vi "Setpoint Status.vi"(8 "error in (no error)":errorcluster, 10 "Output (1:1)":u16(ring)=1 items=["1"=1, "2"=2], 11 "VISA resource name":refnum<visa-resource-name>) -> (0 "error out":errorcluster, 2 "Setpoint":dbl format="%.4f", 3 "VISA resource name out":refnum<visa-resource-name>)   [LabVIEW 2014, in "Lake Shore 335.lvlib"]
doc: "Returns the setpoint value for the selected output."
uses:
  Lake Shore 335.lvlib
  Instance           1 23Saved   Setpoint Status .vi
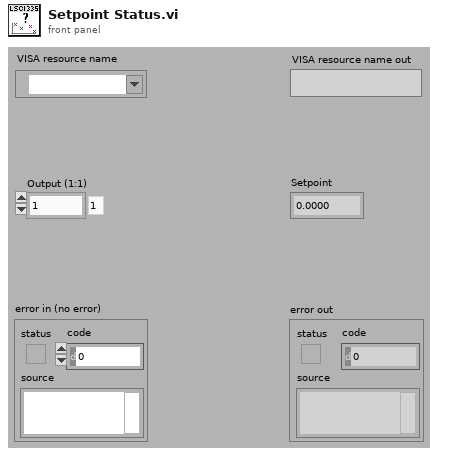
[diagram p1: front panel]
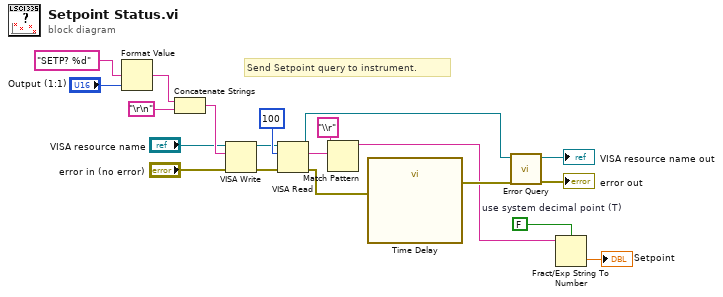
[diagram p0: block diagram]
diagram:
  w20 = FALSE  # use system decimal point (T)
  # "Send Setpoint query to instrument."
  n1 = Format Value(format string="SETP? %d", value (0)="Output (1:1)") -> (output string=w1:string)  [unwired: 1 in]
  n2 = Concatenate Strings(w1, "\r\n") -> (w10:string)
  n3 = VISA Write(VISA resource name="VISA resource name", write buffer=w10, error in (no error)="error in (no error)") -> (VISA resource name out=w14:refnum<visa-resource-name>, error out=w13:errorcluster)  [unwired: 1 out]
  n4 = VISA Read(VISA resource name=w14, byte count=100, error in (no error)=w13) -> (VISA resource name out=w6:refnum<visa-resource-name>, read buffer=w16:string, error out=w12:errorcluster)  [unwired: 1 out]
  n5 = Match Pattern(string=w16, regular expression="\\r") -> (before substring=w4:string)  [unwired: 1 in, 3 out]
  n6 = call "Time Delay"("error in (no error)"=w12) -> ("error out"=w7:errorcluster)  [unwired: 10 in]
  n7 = call "Error Query.vi"("error in (no error)"=w7, "VISA resource name"=w6) -> ("error out"=→"error out":errorcluster, "VISA resource name out"=→"VISA resource name out":refnum<visa-resource-name>)  [unwired: 7 in, 1 out]
  n8 = Fract/Exp String To Number(use system decimal point (T)=w20, string=w4) -> (number=→"Setpoint":dbl)  [unwired: 2 in, 1 out]
